vi "runViWithInput.vi"(6 "valueElement":variant[](array[variant]), 7 "nameElement":string[](array[string]), 8 "error in (no error)":errorcluster, 9 "clusterNameInput":string, 10 "referenceIn":refnum<vi>, 11 "SalProcess in":refnum<class "SalProcess.lvclass">) -> (0 "error out":errorcluster, 2 "referenceOut":refnum<vi>, 3 "SalProcess out":refnum<class "SalProcess.lvclass">)   [LabVIEW 2018, in "SalProcess.lvclass"]
doc: "Run the vi with inputs."
uses:
  SalProcess.lvclass
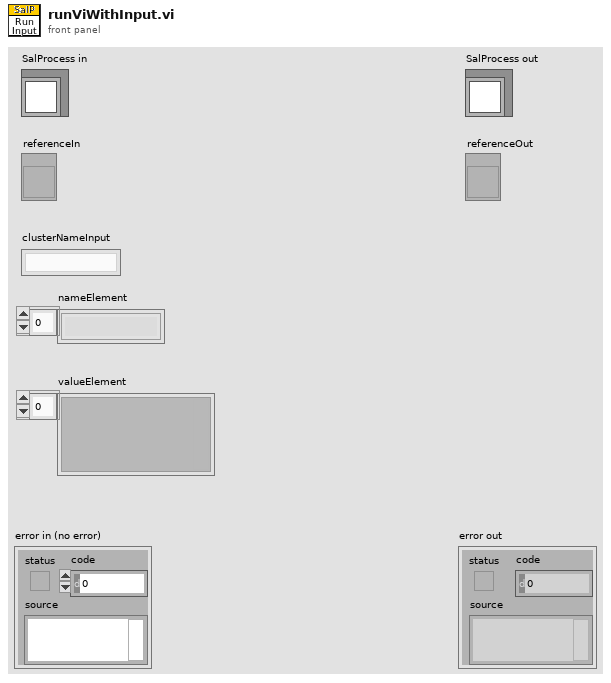
[diagram p1: front panel]
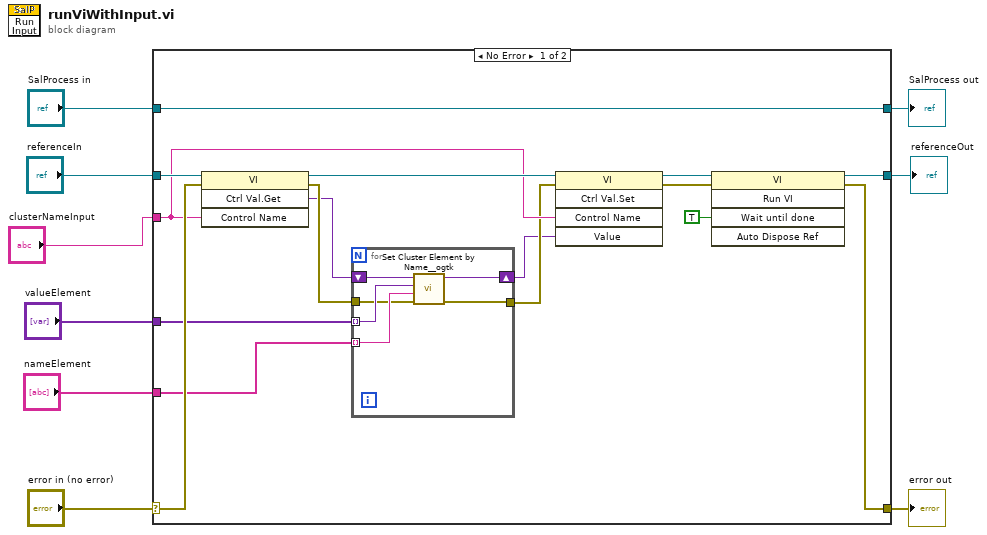
[diagram p0: block diagram]
diagram:
  n1 = case shown="No Error" "error in (no error)" {
    selector: "error in (no error)" -> [w23 w34]
    tunnel: [w12 w34] -> w8
    tunnel: [w25 w33] -> w6
    tunnel: "SalProcess in" -> [w25 w33]
    tunnel: "referenceIn" -> [w24 w32]
    tunnel: "clusterNameInput" -> [w18 _]
    tunnel: "valueElement" -> [w22 _]
    tunnel: "nameElement" -> [w21 _]
    tunnel: [w13 w32] -> w1
    frame No Error {
      n2 = invoke class="VI" method="Ctrl Val.Get"(reference=w24, error in=w23, "Control Name"=w18) -> (reference out=w19:refnum<vi>, error out=w20:errorcluster, "Get Control Value Variant"=w10:variant)  [unwired: 1 in, 1 out]
      n3 = for {
        tunnel: w22 -> [w31] mode=indexing
        tunnel: w21 -> [w30] mode=indexing
        tunnel: w20 -> [w29]
        tunnel: [w28] -> w17
        shift-right: [w26] -> w11
        shift-left: w10 -> [w27]
        n4 = call <userlib>:"Set Cluster Element by Name__ogtk.vi"("error in (no error)"=w29, "Element Name (\"\": New Element Data Name)"=w30, "New Element Value"=w31, "Cluster"=w27) -> ("error out"=w28:errorcluster, "VCluster out"=w26:variant)  [unwired: 5 in, 1 out]
      }
      n5 = invoke class="VI" method="Ctrl Val.Set"(reference=w19, error in=w17, "Control Name"=w18, "Value"=w11) -> (reference out=w15:refnum<vi>, error out=w14:errorcluster)  [unwired: 1 in, 3 out]
      n6 = invoke class="VI" method="Run VI"(reference=w15, error in=w14, "Wait until done"=TRUE ("Wait Until Done")) -> (reference out=w13:refnum<vi>, error out=w12:errorcluster)  [unwired: 2 in, 3 out]
    }
    frame Error {
    }
  }
  "error out" <- w8
  "SalProcess out" <- w6
  "referenceOut" <- w1
